vi "LJM logger open any if device not open.vi"(8 "error in":errorcluster, 9 "Open Config Identifier":string, 10 "Open Config Connection Type":string, 11 "Open Config DeviceType":string) -> (0 "error out":errorcluster, 1 "Open Configs":T2, 2 "Currently Opened Device Params":T1={"Device Type"="ANY", "Connection Type"="ANY", "Serial Number"=0}, 3 "Handle Out":i32)   [LabVIEW 2026]
uses:
  Common Logger Controls/Device Open Config Cluster.ctl
  Common Logger Controls/Currently Opened Device Params.ctl
panel:
  # "Prompts the user to do an \"Open Any\" call if there is an error opening\na device using the input open parameters."
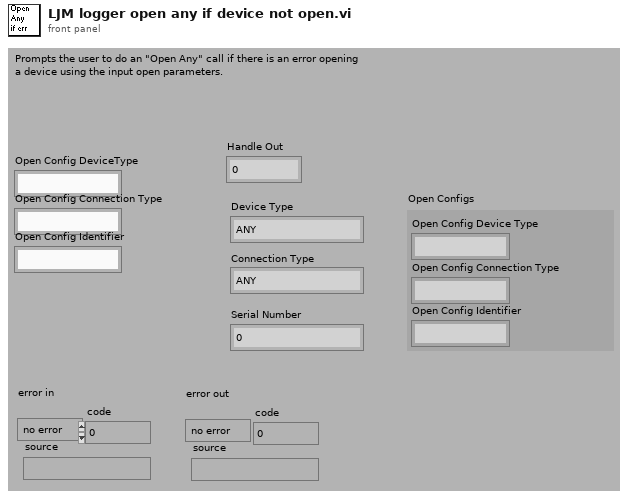
[diagram p1: front panel]
types:
  T1 = typedef "Currently Opened Device Params.ctl" = cluster{"Device Type":string, "Connection Type":string, "Serial Number":i32}
  T2 = typedef "Device Open Config Cluster.ctl" = cluster{"Open Config Device Type":string, "Open Config Connection Type":string, "Open Config Identifier":string}
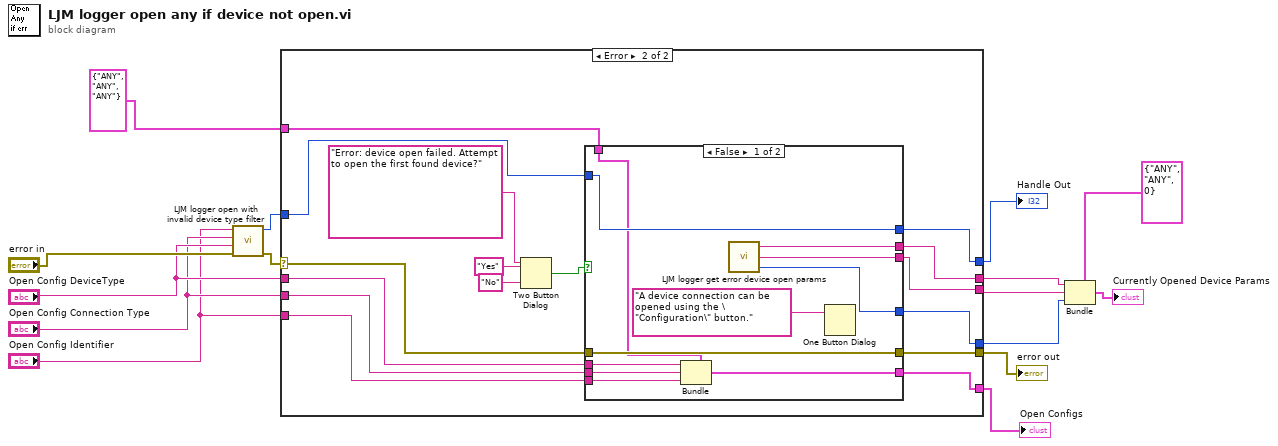
[diagram p0: block diagram]
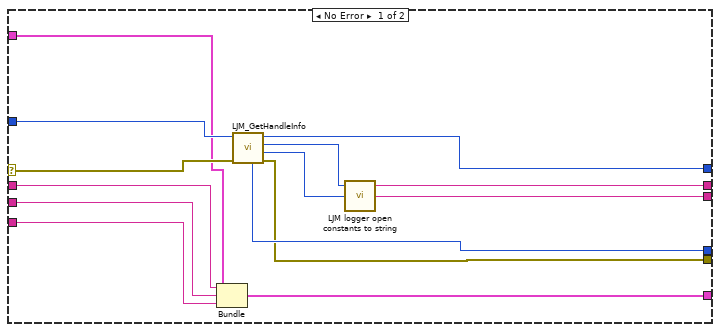
[diagram p2: hidden frame]
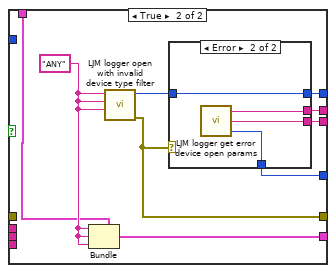
[diagram p3: hidden frame]
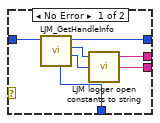
[diagram p4: hidden frame]
diagram:
  n1 = call "LJM logger open with invalid device type filter.vi"("error in"="error in", "DeviceType"="Open Config DeviceType", "ConnectionType"="Open Config Connection Type", "Identifier"="Open Config Identifier") -> ("error out"=w12:errorcluster, "Handle"=w11:i32)  [unwired: 2 in]
  n2 = case shown="Error" w12 {
    selector: w12 -> [w22 w35]
    tunnel: [w27 w44] -> w15
    tunnel: [w29 w42] -> w3
    tunnel: [w28 w41] -> w2
    tunnel: [w21 w43] -> w14
    tunnel: [w24 w45] -> w1
    tunnel: w11 -> [w23 w31]
    tunnel: "Open Config DeviceType" -> [w18 w34]
    tunnel: "Open Config Connection Type" -> [w19 w33]
    tunnel: "Open Config Identifier" -> [w20 w32]
    tunnel: [w17 w40] -> w6
    tunnel: T2 {"Open Config Device Type"="ANY", "Open Config Connection Type"="ANY", "Open Config Identifier"="ANY"} ("Open Configs") -> [w16 w30]
    frame No Error {
      n3 = Bundle(cluster=w16, "Open Config Device Type"=w18, "Open Config Connection Type"=w19, "Open Config Identifier"=w20) -> (w17:T2)
      n4 = call "LJM_GetHandleInfo.vi"("error in"=w22, "Handle In"=w23) -> ("error out"=w21:errorcluster, "ConnectionType"=w25:i32, "DeviceType"=w26:i32, "Handle Out"=w27:i32, "SerialNumber"=w24:i32)  [unwired: 2 in, 3 out]
      n5 = call "LJM logger open constants to string.vi"("ConnType"=w25, "DevType"=w26) -> ("ConnTypeString"=w28:string, "DevTypeString"=w29:string)  [unwired: 2 in]
    }
    frame Error {
      n6 = Two Button Dialog(message="Error: device open failed. Attempt to open the first found device?", 1:"No" ("F button name (\"Cancel\")"), 2:"Yes" ("T button name (\"OK\")")) -> (T button?=w36:bool)
      n7 = case shown="False" w36 {
        tunnel: [w48 w65] -> w45
        tunnel: [w51 w64] -> w44
        tunnel: [w56 w63] -> w43
        tunnel: [w50 w62] -> w42
        tunnel: [w49 w61] -> w41
        tunnel: [w55 w60] -> w40
        tunnel: w35 -> [w56 _]
        tunnel: w34 -> [w54 _]
        tunnel: w33 -> [w53 _]
        tunnel: w32 -> [w52 _]
        tunnel: w31 -> [w51 _]
        tunnel: w30 -> [w46 w57]
        frame False {
          n8 = Bundle(cluster=w46, "Open Config Device Type"=w54, "Open Config Connection Type"=w53, "Open Config Identifier"=w52) -> (w55:T2)
          n9 = call "LJM logger get error device open params.vi"() -> ("Serial Number"=w48:i32, "Connection Type"=w49:string, "Device Type"=w50:string)
          n10 = One Button Dialog(message="A device connection can be opened using the \"Configuration\" button.") -> ()  [unwired: 1 in, 1 out]
        }
        frame True {
          w58 = "ANY"
          n11 = Bundle(cluster=w57, "Open Config Device Type"=w58, "Open Config Connection Type"=w58, "Open Config Identifier"=w58) -> (w60:T2)
          n12 = call "LJM logger open with invalid device type filter.vi"("DeviceType"=w58, "ConnectionType"=w58, "Identifier"=w58) -> ("error out"=w63:errorcluster, "Handle"=w59:i32)  [unwired: 3 in]
          n13 = case shown="Error" w63 {
            tunnel: [w72 w73] -> w65
            tunnel: w59 -> [w71 w76]
            tunnel: [w70 w76] -> w64
            tunnel: [w67 w75] -> w62
            tunnel: [w66 w74] -> w61
            frame No Error {
              n14 = call "LJM_GetHandleInfo.vi"("Handle In"=w71) -> ("ConnectionType"=w68:i32, "DeviceType"=w69:i32, "Handle Out"=w70:i32, "SerialNumber"=w72:i32)  [unwired: 3 in, 4 out]
              n15 = call "LJM logger open constants to string.vi"("ConnType"=w68, "DevType"=w69) -> ("ConnTypeString"=w66:string, "DevTypeString"=w67:string)  [unwired: 2 in]
            }
            frame Error {
              n16 = call "LJM logger get error device open params.vi"() -> ("Serial Number"=w73:i32, "Connection Type"=w74:string, "Device Type"=w75:string)
            }
          }
        }
      }
    }
  }
  "Handle Out" <- w15
  "error out" <- w14
  "Open Configs" <- w6
  n17 = Bundle(cluster=T1 {"Device Type"="ANY", "Connection Type"="ANY", "Serial Number"=0} ("Currently Opened Device Params"), "Device Type"=w3, "Connection Type"=w2, "Serial Number"=w1) -> (→"Currently Opened Device Params":T1)
